vi "AddMeasurement.vi"(7 "measurement-group-id":u16, 8 "error in (no error)":errorcluster, 9 "instrument measure":sgl, 10 "reference measure":sgl, 11 "ByteGSAPIBase in":refnum<class "ByteQXAPIBase.lvclass">) -> (0 "error out":errorcluster, 2 "measurement data":T1, 3 "ByteGSAPIBase out":refnum<class "ByteQXAPIBase.lvclass">)   [LabVIEW 2019, in "ByteQXWebAPI.lvlib" / "ByteQXAPIBase.lvclass"]
doc: "Upload a measurement for an instrument"
uses:
  ByteQXAPIBase.lvclass
  MeasurementResData.ctl
  <vilib>/Bytelabs/ByteREST/ByteRESTClass/ByteRESTBase/HTTP/Status_Code.ctl
  AddMeasurementReqData.ctl
  Private/module.ctl
  ByteQXAPIBase.lvclass/ByteQXAPIBase.ctl
  <vilib>/Bytelabs/ByteREST/ByteRESTClass/ByteRESTBase/RESTBase.lvclass
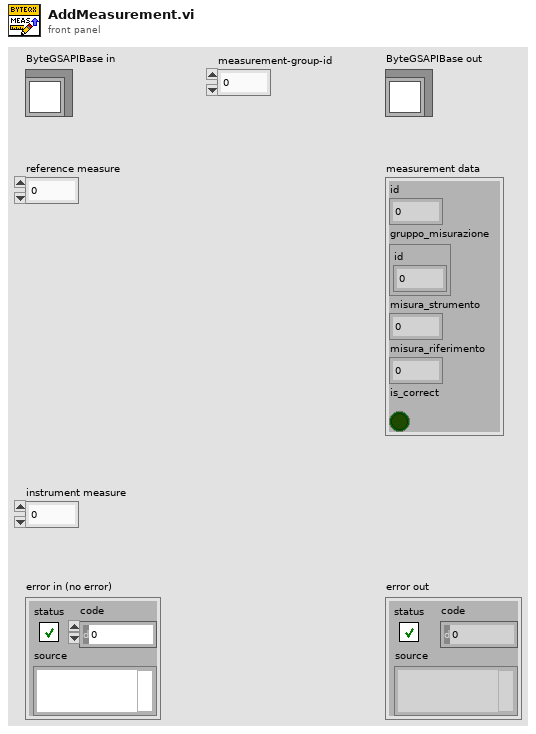
[diagram p1: front panel]
types:
  T1 = typedef "ByteQXWebAPI.lvlib/ByteQXAPIBase.lvclass/MeasurementResData.ctl" = cluster{"id":i32, "gruppo_misurazione":cluster{"id":i32}, "misura_strumento":dbl, "misura_riferimento":dbl, "is_correct":bool}
  T2 = typedef "ByteQXWebAPI.lvlib/ByteQXAPIBase.lvclass/module.ctl" = enum16{"gs", "tms"}
  T3 = typedef "ByteQXWebAPI.lvlib/ByteQXAPIBase.lvclass/AddMeasurementReqData.ctl" = cluster{"misura_strumento":sgl, "misura_riferimento":sgl, "gruppo_misurazione":cluster{"id":i32}}
  T4 = typedef "ByteREST.lvlib/RESTBase.lvclass/Status_Code.ctl" = u16
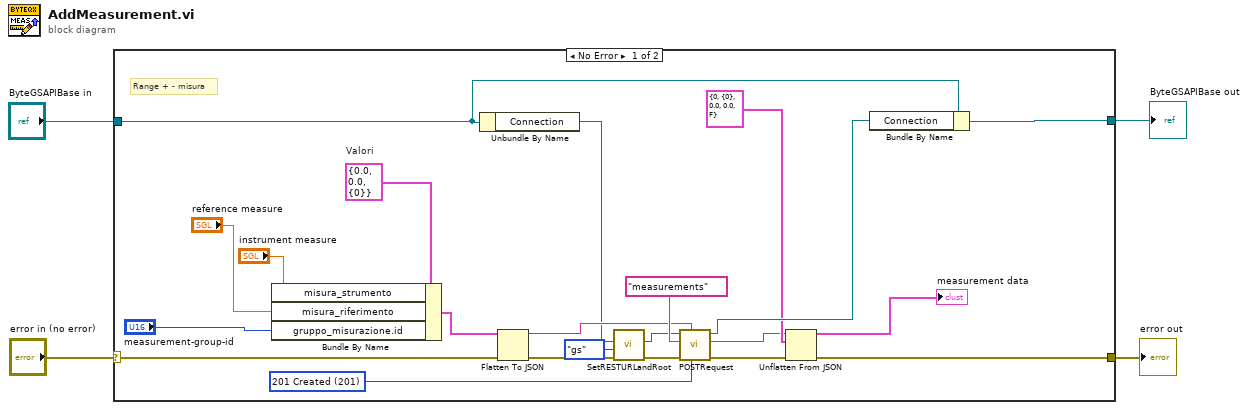
[diagram p0: block diagram]
diagram:
  n1 = case shown="No Error" "error in (no error)" {
    selector: "error in (no error)" -> [w20 w28]
    tunnel: [w15 w28] -> w3
    tunnel: [w25 w27] -> w1
    tunnel: "ByteGSAPIBase in" -> [w26 w27]
    frame No Error {
      w21 = T3 {"misura_strumento"=0.0, "misura_riferimento"=0.0, "gruppo_misurazione"={"id"=0}}  # Valori
      w22 = T4 201 items=["200 OK"=200, "201 Created"=201, "400 Bad Request"=400, "401 Unauthorized"=401, "403 Forbidden"=403, "404 Not Found"=404, "405 Method Not Allowed"=405, "406 Not Acceptable"=406, "500 Internal Server Error"=500] ("expected response")
      # "Range + - misura"
      n2 = Bundle By Name(cluster=w21, "misura_strumento"="instrument measure", "misura_riferimento"="reference measure", "gruppo_misurazione.id"="measurement-group-id") -> (w19:T3)
      n3 = Unbundle By Name(w26) -> ("Connection"=w7:refnum<class "RESTBase.lvclass">)
      n4 = Flatten To JSON(anything=w19, error in (no error)=w20) -> (JSON string=w17:string, 11:w9:errorcluster)  [unwired: 1 in]
      n5 = call "SetRESTURLandRoot.vi"("error in (no error)"=w9, "module"=module."gs", "ByteREST in"=w7) -> ("error out"=w8:errorcluster, "ByteREST out"=w6:refnum<class "RESTBase.lvclass">)  [unwired: 7 in]
      n6 = call-dynamic "POSTRequest.vi"("expected response"=w22, "Body in"=w17, "error in (no error)"=w8, "Request"="measurements", "ByteRESTBase in"=w6) -> ("error out"=w10:errorcluster, "Body"=w11:string, "ByteRESTBase out"=w24:refnum<class "RESTBase.lvclass">)  [unwired: 3 in, 1 out]
      n7 = Unflatten From JSON(JSON string=w11, type and defaults=T1 {"id"=0, "gruppo_misurazione"={"id"=0}, "misura_strumento"=0.0, "misura_riferimento"=0.0, "is_correct"=FALSE}, error in (no error)=w10) -> (value=→"measurement data":T1, error out=w15:errorcluster)  [unwired: 4 in]
      n8 = Bundle By Name(cluster=w26, "Connection"=w24) -> (w25:refnum<class "ByteQXAPIBase.lvclass">)
    }
    frame Error {
    }
  }
  "error out" <- w3
  "ByteGSAPIBase out" <- w1
